vi "RUNfast_derated2.vi"(0 "LWSR":refnum<class "Web Request.lvclass">, 11 "transfer_derate_slope":dbl=-5.2 format="%#_13g", 13 "transfer_derate_base":dbl=350.0 format="%#_13g") -> (7 "GUID":string, 8 "run_order":string, 9 "end_time":string, 10 "tau_mean":dbl format="%0.2f", 12 "tau_std":dbl format="%0.2f", 15 "start_time":string, 16 "Cond (mS) 2":dbl format="%.4g", 17 "Temp (C) 2":dbl format="%#.2g", 19 "transfer_derate":dbl, 21 "viscometer_RPM_end":dbl, 24 "Palmsens-VI-time":dbl, 25 "density (g/mL)":dbl format="%#.4g", 27 "cP_mean":dbl format="%0.3f")   [LabVIEW 2019]
uses:
  <vilib>/wsapi/Web Request.lvclass
  <vilib>/Utility/file.llb/Read Delimited Spreadsheet (string).vi
  <vilib>/Utility/file.llb/Write Delimited Spreadsheet (DBL).vi
panel:
  out "visc_RPM_start":dbl
  out "Retain?":bool
  out "retain_valve":i32
  out "Ohms":dbl
  out "Hz":dbl
  out "mix":timestamp
  out "transfer_viscosity":dbl format="%.2f"
  out "mix-time":u32
  out "Pre-Prime Valve#":i32
  out "preprime_valve":string
  out "Evaluation ET (s)":dbl
  out "start time":timestamp
  out "Viscometer ET (s)":dbl
  out "xfer1":timestamp
  out "debubble":timestamp
  out "fill visc":timestamp
  out "start visc":timestamp
  out "cond2":timestamp
  out "density":timestamp
  out "clear":timestamp
  out "dose":timestamp
  out "empty visc":timestamp
  out "runout":timestamp
  out "Open-Air Valve#":i32
  out "open_valve":string
  out "Chemical, volume (uL) ,valve position":string[][](array[string])=[["", "", "", "30"]]
  out "Splits":i32=4
  out "Constituents":i32=1
  out "run type":string
  out "run ID":string
  out "inventory":string
  out "postdata":string
  out "request method":string
  out "request URI":string
  out "content type":string
  out "remote address":string
  out "Pump2_uL/stroke_":dbl
  out "Pump1_uL/stroke_":dbl
  in  "Pump2_uL/stroke":dbl=6.61
  in  "Pump1_uL/stroke":dbl=5.0
  in  "Viscosity?":bool=TRUE
  out "Background":cluster{"Y":dbl[], "Y":dbl[]}[](graph)
  in  "Spectra?":bool
  out "Baseline Spectrum":cluster{"Y":dbl[], "Y":dbl[]}[](graph)
  out "Ingredient#":i32
  out "RPM":i32
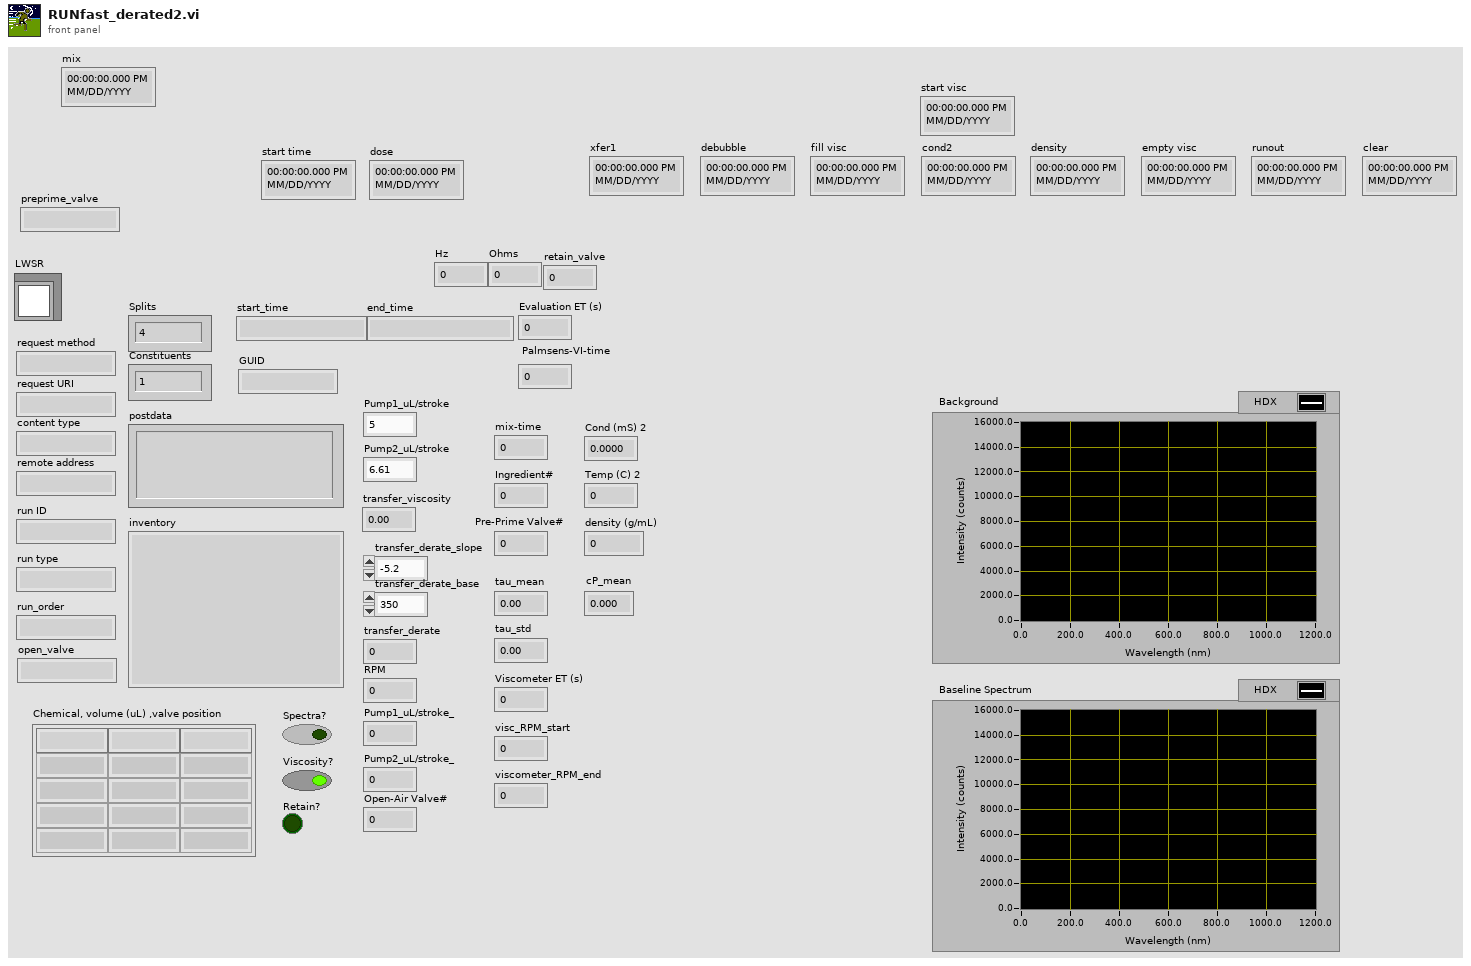
[diagram p1: front panel]
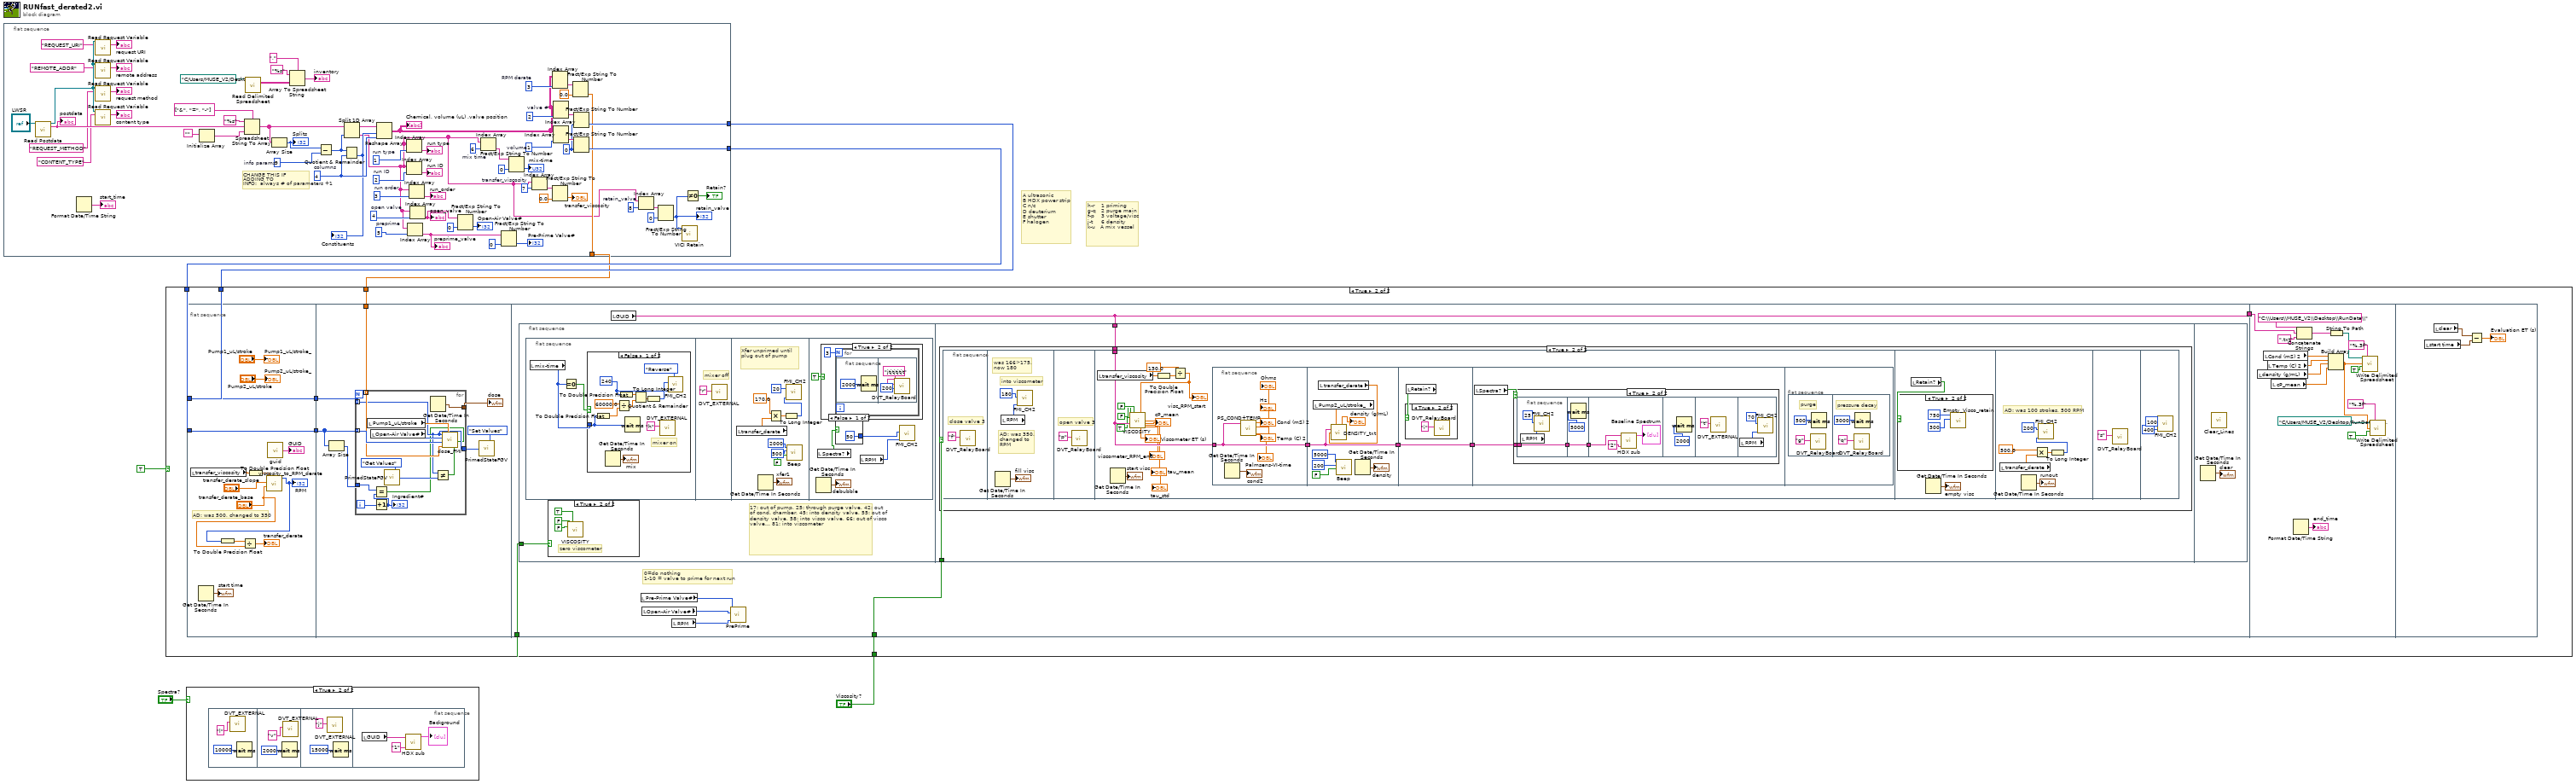
[diagram p0: block diagram]
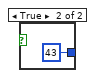
[diagram p4: hidden frame]
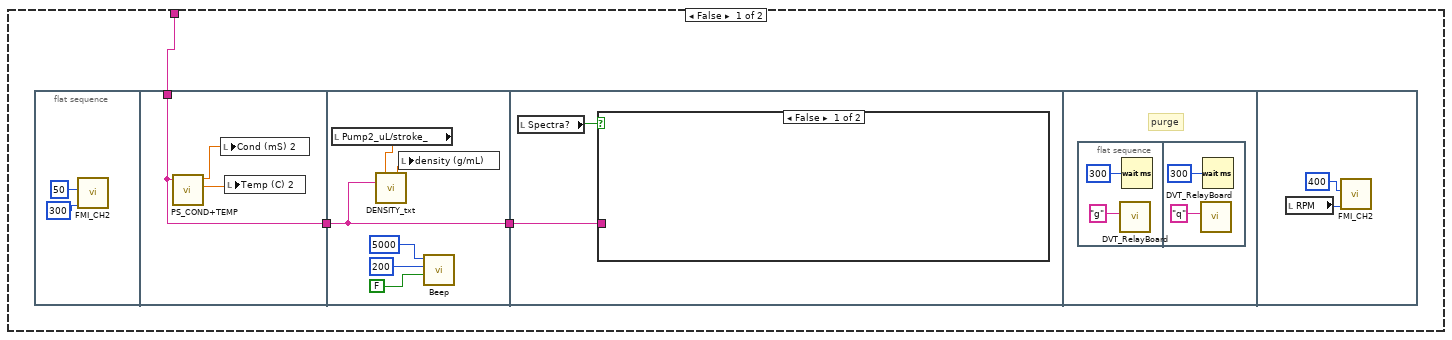
[diagram p7: hidden frame]
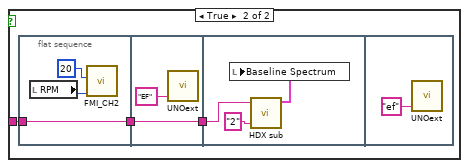
[diagram p8: hidden frame]
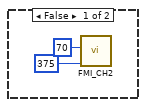
[diagram p10: hidden frame]
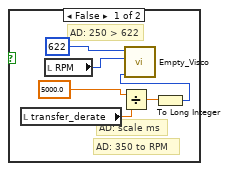
[diagram p11: hidden frame]
diagram:
  # "h-r    1 priming\ng-q   2 purge main\nf-p    3 voltage/visc\nj-t     6 density\nk-u   A mix vessel"
  # "A ultrasonic\nB HDX power strip\nC n/c\nD deuterium\nE shutter\nF halogen"
  n1 = flat-sequence {
    tunnel: [w72] -> w4
    tunnel: [w69] -> w3
    tunnel: [w25] -> w2
    frame #0 {
      w12 = 8  # retain_valve
      w16 = 7  # transfer_viscosity
      w20 = 6  # mix time
      w24 = 5  # preprime
      w28 = 3  # RPM derate
      w30 = 0 ("default (0 DBL)")
      w34 = 4  # open valve
      w54 = 3  # run order
      w57 = 2  # run ID
      w58 = 1  # run type
      w60 = 9  # info params
      w64 = 4  # columns
      w71 = 2  # valve #
      w74 = 1  # volume
      # "CHANGE THIS IF\nADDING TO \nINFO:  always # of parameters +1"
      n2 = call <vilib>:"Read Postdata.vi"("LabVIEW Web Service Request"="LWSR") -> ("LabVIEW Web Service Request out"=w41:refnum<class "Web Request.lvclass">, "postdata"=w47:string)  [unwired: 12 in, 1 out]
      "postdata" <- w47
      n3 = Format Date/Time String() -> (date/time string=→"start_time":string)  [unwired: 3 in]
      n4 = call <vilib>:"Read Request Variable.vi"("LabVIEW Web Service Request"=w41, "variable name"="REQUEST_URI" ("request uri")) -> ("value"=→"request URI":string)  [unwired: 11 in, 2 out]
      n5 = call <vilib>:"Read Request Variable.vi"("LabVIEW Web Service Request"=w41, "variable name"="REMOTE_ADDR" ("remote address")) -> ("value"=→"remote address":string)  [unwired: 11 in, 2 out]
      n6 = call <vilib>:"Read Request Variable.vi"("LabVIEW Web Service Request"=w41, "variable name"="REQUEST_METHOD" ("request method")) -> ("value"=→"request method":string)  [unwired: 11 in, 2 out]
      n7 = call <vilib>:"Read Request Variable.vi"("LabVIEW Web Service Request"=w41, "variable name"="CONTENT_TYPE" ("content type")) -> ("value"=→"content type":string)  [unwired: 11 in, 2 out]
      n8 = Initialize Array("") -> (w66:string[])  [unwired: 1 in]
      n9 = Spreadsheet String To Array(delimiter (Tab)=string[] ["&", "=", "-"], format string="%s", spreadsheet string=w47, array type (2D Dbl)=w66) -> (array=w59:string[])
      n10 = call-poly <vilib>:"Read Delimited Spreadsheet.vi"("file path (dialog if empty)"=path "C:/Users/MUSE_V2/Desktop/CLIO/Public Content/inventory.csv") -> ("all rows"=w51:string[][])  [unwired: 9 in, 5 out]
      n11 = Array Size(array=w59) -> (size(s)=w61:i32)
      "Splits" <- w61
      n12 = Array To Spreadsheet String(delimiter (Tab)=",", array=w51, 3:"%s" ("format string")) -> (spreadsheet string=→"inventory":string)
      n13 = Subtract(x=w61, y=w60) -> (x-y=w46:i32)
      n14 = Split 1D Array(array=w59, index=w46) -> (first subarray=w52:string[], second subarray=w9:string[])
      n15 = Quotient & Remainder(x=w46, y=w64) -> (floor(x/y)=w63:i32)  [unwired: 1 out]
      "Constituents" <- w63
      n16 = Reshape Array(w52, w63, w64) -> (w27:string[][])
      "Chemical, volume (uL) ,valve position" <- w27
      n17 = Index Array(array=w9, index=w58) -> (element=→"run type":string)
      n18 = Index Array(array=w9, index=w57) -> (element=→"run ID":string)
      n19 = Index Array(array=w9, index=w24) -> (element=w22:string)
      "preprime_valve" <- w22
      n20 = Index Array(array=w9, index=w54) -> (element=→"run_order":string)
      n21 = Index Array(array=w9, index=w34) -> (element=w33:string)
      "open_valve" <- w33
      n22 = Fract/Exp String To Number(string=w33, default (0 dbl)=0 ("default (0 DBL)")) -> (number=→"Open-Air Valve#":i32)  [unwired: 2 in, 1 out]
      n23 = Index Array(array=w9, index=w20) -> (element=w19:string)
      n24 = Fract/Exp String To Number(string=w22, default (0 dbl)=0 ("default (0 DBL)")) -> (number=→"Pre-Prime Valve#":i32)  [unwired: 2 in, 1 out]
      n25 = Fract/Exp String To Number(string=w19, default (0 dbl)=u32 0 ("default (0 DBL)")) -> (number=→"mix-time":u32)  [unwired: 2 in, 1 out]
      n26 = Index Array(array=w9, index=w16) -> (element=w15:string)
      n27 = Index Array(array=w27, index (col)=w28) -> (element=w29:string[])  [unwired: 1 in]
      n28 = Fract/Exp String To Number(string=w15, default (0 dbl)=0.0 ("default (0 DBL)")) -> (number=→"transfer_viscosity":dbl)  [unwired: 2 in, 1 out]
      n29 = Index Array(array=w27, index (col)=w71) -> (element=w70:string[])  [unwired: 1 in]
      n30 = Index Array(array=w27, index (col)=w74) -> (element=w73:string[])  [unwired: 1 in]
      n31 = Fract/Exp String To Number(string=w29, default (0 dbl)=0.0 ("default (0 DBL)")) -> (number=w25:dbl[])  [unwired: 2 in, 1 out]
      n32 = Fract/Exp String To Number(string=w70, default (0 dbl)=w30) -> (number=w69:i32[])  [unwired: 2 in, 1 out]
      n33 = Fract/Exp String To Number(string=w73, default (0 dbl)=w30) -> (number=w72:i32[])  [unwired: 2 in, 1 out]
      n34 = Index Array(array=w9, index=w12) -> (element=w11:string)
      n35 = Fract/Exp String To Number(string=w11, default (0 dbl)=0 ("default (0 DBL)")) -> (number=w8:i32)  [unwired: 2 in, 1 out]
      "retain_valve" <- w8
      n36 = call "VICI Retain.vi"("RequestedValve#"=w8) -> ()  [unwired: 2 in, 3 out]
      n37 = Not Equal To 0?(x=w8) -> (x != 0?=→"Retain?":bool)
    }
  }
  n38 = case shown="True" TRUE {
    tunnel: "Viscosity?" -> [_ w78]
    tunnel: w4 -> [_ w77]
    tunnel: w3 -> [_ w76]
    tunnel: w2 -> [_ w75]
    frame False {
    }
    frame True {
      n39 = flat-sequence {
        tunnel: [w91] -> w81
        tunnel: [w90] -> w80
        tunnel: w77 -> [w91]
        tunnel: w76 -> [w90]
        tunnel: w81 -> [w96]
        tunnel: w80 -> [w101]
        tunnel: w75 -> [w100]
        tunnel: [w118] -> w79
        tunnel: w78 -> [w120]
        tunnel: w78 -> [w119]
        tunnel: w79 -> [w289]
        frame #0 {
          # "AD: was 500, changed to 350"
          n40 = local read "transfer_viscosity"() -> (w86:dbl)
          n41 = Get Date/Time In Seconds() -> (seconds since 1Jan1904=→"start time":timestamp)
          n42 = To Double Precision Float(number=w86) -> (double precision float=w87:dbl)
          n43 = call "viscosity_to_RPM_derate.vi"("base RPM"="transfer_derate_base", "slope"="transfer_derate_slope", "viscosity (cP)"=w87) -> ("output_RPM"=w85:i32)  [unwired: 7 in]
          "RPM" <- w85
          n44 = To Double Precision Float(number=w85) -> (double precision float=w84:dbl)
          n45 = Divide(x=w84, y="transfer_derate_base") -> (x/y=→"transfer_derate":dbl)
          n46 = call "guid.vi"() -> ("GUID String"=→"GUID":string)  [unwired: 1 in]
          "Pump1_uL/stroke_" <- "Pump1_uL/stroke"
          "Pump2_uL/stroke_" <- "Pump2_uL/stroke"
        }
        frame #1 {
          n47 = Array Size(array=w96) -> (size(s)=w95:i32)
          n48 = for {
            tunnel: w101 -> [w107] mode=indexing
            tunnel: w96 -> [w114] mode=indexing
            tunnel: w100 -> [w112] mode=indexing
            tunnel: [w107] -> w99
            tunnel: [w110] -> w97
            tunnel: w95 -> [w105]
            i -> [w104]
            n49 = local read "Pump1_uL/stroke"() -> (w111:dbl)
            n50 = local read "Open-Air Valve#"() -> (w113:i32)
            n51 = Increment(x=w104) -> (x+1=w102:i32)
            "Ingredient#" <- w102
            n52 = Equal?(x=w105, y=w102) -> (x = y?=w103:bool)
            n53 = call "PrimedStateFGV.vi"("Enum"=enum16{"Set Values", "Set Time", "Get Values"}."Get Values") -> ("LastValve_read"=w106:i32)  [unwired: 13 in, 1 out]
            n54 = Get Date/Time In Seconds() -> (seconds since 1Jan1904=w110:timestamp)
            n55 = Not Equal?(x=w107, y=w106) -> (x != y?=w108:bool)
            n56 = call "dose_FMI.vi"("Prime?"=w108, "Final Ingredient?"=w103, "uL/stroke"=w111, "RPM Derate"=w112, "Volume (uL)"=w114, "OpenValve#"=w113, "RequestedValve#"=w107) -> ()  [unwired: 3 in]
          }
          "dose" <- w97
          n57 = call "PrimedStateFGV.vi"("Enum"=enum16{"Set Values", "Set Time", "Get Values"}."Set Values", "LastValve_write"=w99) -> ()  [unwired: 12 in, 2 out]
        }
        frame #2 {
          # "0=do nothing\n1-10 = valve to prime for next run"
          n58 = flat-sequence {
            tunnel: w119 -> [w121]
            tunnel: w118 -> [w160]
            tunnel: w120 -> [w159]
            frame #0 {
              # "17: out of pump, 25: through purge valve, 42: out of cond. chamber, 45: into density valve, 55: out of density valve, 58: into visco valve, 66: out of visco valve... 81: into viscometer"
              n59 = flat-sequence {
                frame #0 {
                  n60 = local read "mix-time"() -> (w122:u32)
                  n61 = Equal To 0?(x=w122) -> (x = 0?=w123:bool)
                  n62 = case shown="False" w123 {
                    tunnel: w122 -> [w125 _]
                    frame False {
                      w128 = 240 ("RPM")
                      # "mixer on"
                      n63 = To Double Precision Float(number=w125) -> (double precision float=w126:dbl)
                      n64 = Get Date/Time In Seconds() -> (seconds since 1Jan1904=→"mix":timestamp)
                      n65 = Divide(x=60000.0, y=w126) -> (x/y=w131:dbl)
                      n66 = To Double Precision Float(number=w128) -> (double precision float=w127:dbl)
                      n67 = Wait (ms)(milliseconds to wait=w125) -> ()  [unwired: 1 out]
                      n68 = Quotient & Remainder(x=w127, y=w131) -> (floor(x/y)=w129:dbl)  [unwired: 1 out]
                      n69 = To Long Integer(number=w129) -> (32bit integer=w130:i32)
                      n70 = call "DVT_EXTERNAL.vi"("write buffer"="h") -> ()  [unwired: 3 in, 3 out]
                      n71 = call "FMI_CH2.vi"("Direction"=enum16{"Forward", "Reverse"}."Reverse", "RPM"=w128, "Strokes"=w130) -> ()  [unwired: 4 in, 1 out]
                    }
                    frame True {
                    }
                  }
                }
                frame #1 {
                  # "mixer off"
                  n72 = call "DVT_EXTERNAL.vi"("write buffer"="r") -> ()  [unwired: 3 in, 3 out]
                }
                frame #2 {
                  # "Xfer unprimed until plug out of pump"
                  n73 = local read "transfer_derate"() -> (w136:dbl)
                  n74 = Get Date/Time In Seconds() -> (seconds since 1Jan1904=→"xfer1":timestamp)
                  n75 = Multiply(x=170.0 ("RPM"), y=w136) -> (x*y=w139:dbl)
                  n76 = To Long Integer(number=w139) -> (32bit integer=w137:i32)
                  n77 = call "FMI_CH2.vi"("RPM"=w137, "Strokes"=20) -> ()  [unwired: 5 in, 1 out]
                  n78 = call <vilib>:"Beep.vi"("use system alert? (T)"=FALSE, "duration (msec)"=u32 500, "frequency (Hz)"=u32 2000) -> ()  [unwired: 9 in]
                }
                frame #3 {
                  n79 = Get Date/Time In Seconds() -> (seconds since 1Jan1904=→"debubble":timestamp)
                  n80 = local read "Spectra?"() -> (w146:bool)
                  n81 = case shown="True" TRUE {
                    frame False {
                    }
                    frame True {
                      n82 = for {
                        N: 3 -> [_]
                        n83 = flat-sequence {
                          frame #0 {
                            n84 = Wait (ms)(milliseconds to wait=u32 2000) -> ()  [unwired: 1 out]
                          }
                          frame #1 {
                            n85 = call "DVT_RelayBoard.vi"("ms"=u32 200, "write buffer"="jtjtjtjtjt") -> ()  [unwired: 2 in, 3 out]
                          }
                        }
                      }
                    }
                  }
                  n86 = case shown="False" w146 {
                    tunnel: [50 ("Strokes") 43 ("Strokes")] -> w145
                    frame False {
                    }
                    frame True {
                    }
                  }
                  n87 = local read "RPM"() -> (w147:i32)
                  n88 = call "FMI_CH2.vi"("RPM"=w147, "Strokes"=w145) -> ()  [unwired: 5 in, 1 out]
                }
              }
              n89 = case shown="True" w121 {
                frame False {
                }
                frame True {
                  # "zero viscometer"
                  n90 = call "VISCOSITY.vi"("SPIN (F)"=FALSE, "Zero? (T)"=TRUE ("Zero?"), "LogData? (T)"=FALSE ("LogData?")) -> ()  [unwired: 6 in, 7 out]
                }
              }
            }
            frame #1 {
              n91 = case shown="True" w159 {
                tunnel: w160 -> [w161 w195]
                frame False {
                  n92 = flat-sequence {
                    tunnel: [w166] -> w162
                    tunnel: w161 -> [w166]
                    tunnel: [w171] -> w163
                    tunnel: w162 -> [w171]
                    tunnel: w163 -> [w176]
                    frame #0 {
                      n93 = call "FMI_CH2.vi"("RPM"=300, "Strokes"=50) -> ()  [unwired: 5 in, 1 out]
                    }
                    frame #1 {
                      n94 = call "PS_COND+TEMP.vi"("GUID"=w166) -> ("Cond (mS)"=w168:dbl, "Temp (C)"=w167:dbl)  [unwired: 1 in, 7 out]
                      n95 = local write "Cond (mS) 2"(w168) -> ()
                      n96 = local write "Temp (C) 2"(w167) -> ()
                    }
                    frame #2 {
                      n97 = local read "Pump2_uL/stroke_"() -> (w170:dbl)
                      n98 = call "DENSITY_txt.vi"("uL/stroke"=w170, "GUID"=w171) -> ("density (g/mL)"=w169:dbl)  [unwired: 7 in, 6 out]
                      n99 = local write "density (g/mL)"(w169) -> ()
                      n100 = call <vilib>:"Beep.vi"("use system alert? (T)"=FALSE, "duration (msec)"=u32 200, "frequency (Hz)"=u32 5000) -> ()  [unwired: 9 in]
                    }
                    frame #3 {
                      n101 = local read "Spectra?"() -> (w175:bool)
                      n102 = case shown="False" w175 {
                        tunnel: w176 -> [_ w179]
                        frame False {
                        }
                        frame True {
                          n103 = flat-sequence {
                            tunnel: w179 -> [w182]
                            tunnel: [w182] -> w177
                            tunnel: [w184] -> w178
                            tunnel: w177 -> [w184]
                            tunnel: w178 -> [w187]
                            frame #0 {
                              n104 = local read "RPM"() -> (w181:i32)
                              n105 = call "FMI_CH2.vi"("RPM"=w181, "Strokes"=20) -> ()  [unwired: 5 in, 1 out]
                            }
                            frame #1 {
                              n106 = call "UNOext.vi"("write buffer"="EF") -> ()  [unwired: 2 in, 3 out]
                            }
                            frame #2 {
                              n107 = call "HDX sub.vi"("GUID"=w187, "SCAN#"="2") -> ("Transmission Spectrum"=w185:cluster{"Y":dbl[], "Y":dbl[]}[])  [unwired: 1 in, 3 out]
                              n108 = local write "Baseline Spectrum"(w185) -> ()
                            }
                            frame #3 {
                              n109 = call "UNOext.vi"("write buffer"="ef") -> ()  [unwired: 2 in, 3 out]
                            }
                          }
                        }
                      }
                    }
                    frame #4 {
                      # "purge"
                      n110 = flat-sequence {
                        frame #0 {
                          n111 = call "DVT_RelayBoard.vi"("write buffer"="g") -> ()  [unwired: 3 in, 3 out]
                          n112 = Wait (ms)(milliseconds to wait=u32 300) -> ()  [unwired: 1 out]
                        }
                        frame #1 {
                          n113 = call "DVT_RelayBoard.vi"("write buffer"="q") -> ()  [unwired: 3 in, 3 out]
                          n114 = Wait (ms)(milliseconds to wait=u32 300) -> ()  [unwired: 1 out]
                        }
                      }
                    }
                    frame #5 {
                      n115 = local read "RPM"() -> (w194:i32)
                      n116 = call "FMI_CH2.vi"("RPM"=w194, "Strokes"=400) -> ()  [unwired: 5 in, 1 out]
                    }
                  }
                }
                frame True {
                  n117 = flat-sequence {
                    tunnel: w195 -> [w215]
                    frame #0 {
                      # "close valve 3"
                      n118 = call "DVT_RelayBoard.vi"("write buffer"="f") -> ()  [unwired: 3 in, 3 out]
                    }
                    frame #1 {
                      # "was 166>175, now 180"
                      # "AD: was 350, changed to RPM"
                      # "into viscometer"
                      n119 = Get Date/Time In Seconds() -> (seconds since 1Jan1904=→"fill visc":timestamp)
                      n120 = local read "RPM"() -> (w197:i32)
                      n121 = call "FMI_CH2.vi"("RPM"=w197, "Strokes"=180) -> ()  [unwired: 5 in, 1 out]
                    }
                    frame #2 {
                      # "open valve 3"
                      n122 = call "DVT_RelayBoard.vi"("write buffer"="p") -> ()  [unwired: 3 in, 3 out]
                    }
                    frame #3 {
                      n123 = local read "transfer_viscosity"() -> (w206:dbl)
                      n124 = Get Date/Time In Seconds() -> (seconds since 1Jan1904=→"start visc":timestamp)
                      n125 = To Double Precision Float(number=w206) -> (double precision float=w205:dbl)
                      n126 = Divide(x=130.0, y=w205) -> (x/y=w203:dbl)
                      "visc_RPM_start" <- w203
                      n127 = call "VISCOSITY.vi"("SPIN (F)"=FALSE, "Zero? (T)"=FALSE ("Zero?"), "Startup RPM"=w203, "LogData? (T)"=TRUE, "GUID"=w215) -> ("final_RPM"=→"viscometer_RPM_end":dbl, "cP_mean"=→"cP_mean":dbl, "tau_std"=→"tau_std":dbl, "ET (s)"=→"Viscometer ET (s)":dbl, "tau_mean"=→"tau_mean":dbl)  [unwired: 4 in, 2 out]
                      n128 = flat-sequence {
                        tunnel: w215 -> [w224]
                        tunnel: [w224] -> w212
                        tunnel: [w226] -> w209
                        tunnel: w212 -> [w226]
                        tunnel: w209 -> [w234]
                        tunnel: [w234] -> w208
                        tunnel: w208 -> [w237]
                        frame #0 {
                          n129 = Get Date/Time In Seconds() -> (seconds since 1Jan1904=→"cond2":timestamp)
                          n130 = call "PS_COND+TEMP.vi"("GUID"=w224) -> ("Ohms"=→"Ohms":dbl, "VI-time"=→"Palmsens-VI-time":dbl, "Cond (mS)"=→"Cond (mS) 2":dbl, "Temp (C)"=→"Temp (C) 2":dbl, "Hz"=→"Hz":dbl)  [unwired: 1 in, 4 out]
                        }
                        frame #1 {
                          n131 = local read "Pump2_uL/stroke_"() -> (w228:dbl)
                          n132 = local read "transfer_derate"() -> (w225:dbl)
                          n133 = call "DENSITY_txt.vi"("uL/stroke"=w228, "GUID"=w226, "derate"=w225) -> ("density (g/mL)"=→"density (g/mL)":dbl)  [unwired: 6 in, 6 out]
                          n134 = call <vilib>:"Beep.vi"("use system alert? (T)"=FALSE, "duration (msec)"=u32 200, "frequency (Hz)"=u32 5000) -> ()  [unwired: 9 in]
                          n135 = Get Date/Time In Seconds() -> (seconds since 1Jan1904=→"density":timestamp)
                        }
                        frame #2 {
                          n136 = local read "Retain?"() -> (w233:bool)
                          n137 = case shown="True" w233 {
                            frame False {
                            }
                            frame True {
                              n138 = call "DVT_RelayBoard.vi"("write buffer"="i") -> ()  [unwired: 3 in, 3 out]
                            }
                          }
                        }
                        frame #3 {
                          n139 = local read "Spectra?"() -> (w236:bool)
                          n140 = case shown="True" w236 {
                            tunnel: w237 -> [_ w242]
                            frame False {
                              n141 = call "FMI_CH2.vi"("RPM"=375, "Strokes"=70) -> ()  [unwired: 5 in, 1 out]
                            }
                            frame True {
                              n142 = flat-sequence {
                                tunnel: [w245] -> w241
                                tunnel: w242 -> [w245]
                                tunnel: w241 -> [w247]
                                tunnel: [w247] -> w240
                                tunnel: w240 -> [w249]
                                frame #0 {
                                n143 = local read "RPM"() -> (w243:i32)
                                n144 = call "FMI_CH2.vi"("RPM"=w243, "Strokes"=25) -> ()  [unwired: 5 in, 1 out]
                                }
                                frame #1 {
                                n145 = Wait (ms)(milliseconds to wait=u32 5000) -> ()  [unwired: 1 out]
                                }
                                frame #2 {
                                n146 = call "HDX sub.vi"("GUID"=w249, "SCAN#"="2") -> ("Transmission Spectrum"=→"Baseline Spectrum":cluster{"Y":dbl[], "Y":dbl[]}[])  [unwired: 1 in, 3 out]
                                }
                                frame #3 {
                                n147 = Wait (ms)(milliseconds to wait=u32 2000) -> ()  [unwired: 1 out]
                                }
                                frame #4 {
                                n148 = call "DVT_EXTERNAL.vi"("write buffer"="t") -> ()  [unwired: 3 in, 3 out]
                                }
                                frame #5 {
                                n149 = local read "RPM"() -> (w253:i32)
                                n150 = call "FMI_CH2.vi"("RPM"=w253, "Strokes"=70) -> ()  [unwired: 5 in, 1 out]
                                }
                              }
                            }
                          }
                        }
                        frame #4 {
                          n151 = flat-sequence {
                            frame #0 {
                              # "purge"
                              n152 = call "DVT_RelayBoard.vi"("write buffer"="g") -> ()  [unwired: 3 in, 3 out]
                              n153 = Wait (ms)(milliseconds to wait=u32 500) -> ()  [unwired: 1 out]
                            }
                            frame #1 {
                              # "pressure decay"
                              n154 = call "DVT_RelayBoard.vi"("write buffer"="q") -> ()  [unwired: 3 in, 3 out]
                              n155 = Wait (ms)(milliseconds to wait=u32 3000) -> ()  [unwired: 1 out]
                            }
                          }
                        }
                      }
                    }
                    frame #4 {
                      n156 = local read "Retain?"() -> (w259:bool)
                      n157 = case shown="True" w259 {
                        frame False {
                          # "AD: scale ms"
                          # "AD: 350 to RPM"
                          # "AD: 250 > 622"
                          n158 = local read "transfer_derate"() -> (w261:dbl)
                          n159 = local read "RPM"() -> (w265:i32)
                          n160 = Divide(x=5000.0, y=w261) -> (x/y=w263:dbl)
                          n161 = To Long Integer(number=w263) -> (32bit integer=w262:i32)
                          n162 = call "Empty_Visco.vi"("ms"=w262, "RPM"=w265, "Strokes"=622) -> ()  [unwired: 9 in]
                        }
                        frame True {
                          n163 = call "Empty_Visco_retain.vi"("RPM"=300, "Strokes"=750) -> ()  [unwired: 10 in]
                        }
                      }
                      n164 = Get Date/Time In Seconds() -> (seconds since 1Jan1904=→"empty visc":timestamp)
                    }
                    frame #5 {
                      # "AD: was 100 strokes, 500 RPM"
                      n165 = local read "transfer_derate"() -> (w269:dbl)
                      n166 = Get Date/Time In Seconds() -> (seconds since 1Jan1904=→"runout":timestamp)
                      n167 = Multiply(x=500.0, y=w269) -> (x*y=w271:dbl)
                      n168 = To Long Integer(number=w271) -> (32bit integer=w270:i32)
                      n169 = call "FMI_CH2.vi"("RPM"=w270, "Strokes"=200) -> ()  [unwired: 5 in, 1 out]
                    }
                    frame #6 {
                      n170 = call "DVT_RelayBoard.vi"("write buffer"="s") -> ()  [unwired: 3 in, 3 out]
                    }
                    frame #7 {
                      n171 = call "FMI_CH2.vi"("RPM"=400, "Strokes"=100) -> ()  [unwired: 5 in, 1 out]
                    }
                  }
                }
              }
            }
            frame #2 {
              n172 = Get Date/Time In Seconds() -> (seconds since 1Jan1904=→"clear":timestamp)
              n173 = call "Clear_Lines.vi"() -> ()  [unwired: 12 in]
            }
          }
          n174 = local read "GUID"() -> (w118:string)
          n175 = local read "Pre-Prime Valve#"() -> (w117:i32)
          n176 = local read "Open-Air Valve#"() -> (w116:i32)
          n177 = local read "RPM"() -> (w115:i32)
          n178 = call "PrePrime.vi"("RPM"=w115, "OpenValve#"=w116, "RequestedValve#"=w117) -> ()  [unwired: 5 in]
        }
        frame #3 {
          n179 = local read "density (g/mL)"() -> (w281:dbl)
          n180 = local read "Cond (mS) 2"() -> (w279:dbl)
          n181 = local read "Temp (C) 2"() -> (w280:dbl)
          n182 = local read "cP_mean"() -> (w287:dbl)
          n183 = Format Date/Time String() -> (date/time string=→"end_time":string)  [unwired: 3 in]
          n184 = Concatenate Strings("C:\\Users\\MUSE_V2\\Desktop\\RunData\\", w289, ".txt" ("string")) -> (w291:string)
          n185 = Build Array(w279, w280, w281, w287) -> (w282:dbl[])
          n186 = String To Path(string=w291) -> (path=w288:path)
          n187 = call-poly <vilib>:"Write Delimited Spreadsheet.vi"("file path (dialog if empty)"=w288, "format (%.3f)"="%.3f", "1D data"=w282, "append to file? (new file:F)"=TRUE) -> ()  [unwired: 10 in, 2 out]
          n188 = call-poly <vilib>:"Write Delimited Spreadsheet.vi"("file path (dialog if empty)"=path "C:/Users/MUSE_V2/Desktop/RunData/00_AppendedLog.txt" ("file path (use dialog)"), "format (%.3f)"="%.3f", "1D data"=w282, "append to file? (new file:F)"=TRUE) -> ()  [unwired: 10 in, 2 out]
        }
        frame #4 {
          n189 = local read "start time"() -> (w296:timestamp)
          n190 = local read "clear"() -> (w297:timestamp)
          n191 = Subtract(x=w297, y=w296) -> (x-y=→"Evaluation ET (s)":dbl)
        }
      }
    }
  }
  n192 = case shown="True" "Spectra?" {
    frame False {
    }
    frame True {
      n193 = flat-sequence {
        frame #0 {
          n194 = call "DVT_EXTERNAL.vi"("write buffer"="l") -> ()  [unwired: 3 in, 3 out]
          n195 = Wait (ms)(milliseconds to wait=u32 10000) -> ()  [unwired: 1 out]
        }
        frame #1 {
          n196 = Wait (ms)(milliseconds to wait=u32 2000) -> ()  [unwired: 1 out]
          n197 = call "DVT_EXTERNAL.vi"("write buffer"="v") -> ()  [unwired: 3 in, 3 out]
        }
        frame #2 {
          n198 = call "DVT_EXTERNAL.vi"("write buffer"="j") -> ()  [unwired: 3 in, 3 out]
          n199 = Wait (ms)(milliseconds to wait=u32 15000) -> ()  [unwired: 1 out]
        }
        frame #3 {
          n200 = local read "GUID"() -> (w304:string)
          n201 = call "HDX sub.vi"("GUID"=w304, "SCAN#"="1") -> ("Transmission Spectrum"=→"Background":cluster{"Y":dbl[], "Y":dbl[]}[])  [unwired: 1 in, 3 out]
        }
      }
    }
  }
